vi "o3 49i Serial Data Recording & DECADEv3.2.vi"() -> ()   [LabVIEW 2014]
uses:
  <vilib>/Platform/TimedLoop/XDataNode/timing_clust.ctl
  <vilib>/Platform/TimedLoop/XDataNode/nitl_modes.ctl
  <vilib>/Platform/TimedLoop/XDataNode/wakeup.ctl
  C:/Program Files (x86)/National Instruments/LabVIEW 2014/examples/Data Communication/Network Streams/Simple Network Streams/support/Network Stream Command.ctl
  <vilib>/Utility/error.llb/whitespace.ctl
  <vilib>/Instr/_visa.llb/VISA Configure Serial Port (Instr).vi
  <vilib>/Utility/tcp.llb/UDP Multicast Write-Only Open.vi
  <vilib>/platform/TimedLoop/XDataNode/XDataNode.xnode
  <vilib>/Platform/TimedLoop/XDataNode/XDNodeRunTimeDep.lvlib
panel:
  in  "MFC_1 SLPM set value":dbl
  out "Stop File Write":bool
  out "Default file name":string
  out "error out":errorcluster
  out "V6":bool
  in  "Clear Display\nErrors":bool
  out "Data Processing":bool
  out "Serial Visa Error":errorcluster
  out "SEPTIC TCP Error Out":errorcluster
  out "TCP packet\nSend to SEPTIC":bool
  out "UDP Time Stamp Offset":i32=1
  out "Data Array":string[](array[string])
  out "UDP packet \nstatus":bool
  out "UDP_Out_Error":errorcluster
  out "FISH TCP Error Out":errorcluster
  out "TCP packet\nSend to FISH":bool
  out "TCP Binary Packet":string
  out "Scan from String Error Counter\nfrom process loop":i32
  out "Read Error Counter\nfrom process loop":i32
  in  "milliseconds to wait":u32=330
  in  "ID":string="»"
  in  "VISA resource name":refnum<visa-resource-name>="ASRL6::INSTR"
  out "Data In Array":string[](array[string])
  out "UDP_ASCII_Out":string
  out "UDP_Pack_num":u32
  out "Flight Number":string
  in  "ue9LJ temp":u16
  out "Data String":string
  out "Internal packet":string[](array[string])
  out "RAW DATA":string
  in  "stop":bool
  out "Number of Send & Read Error\nfrom Acquire Loop":i32
  out "Command In":string
  # "o3_conc"
  # "Bench_temp"
  # "pressure"
  # "cell_a_nt"
  # "cell_b_int"
  # "flow_a"
  # "flow_b"
  # "lamp_temp"
  # "flags"
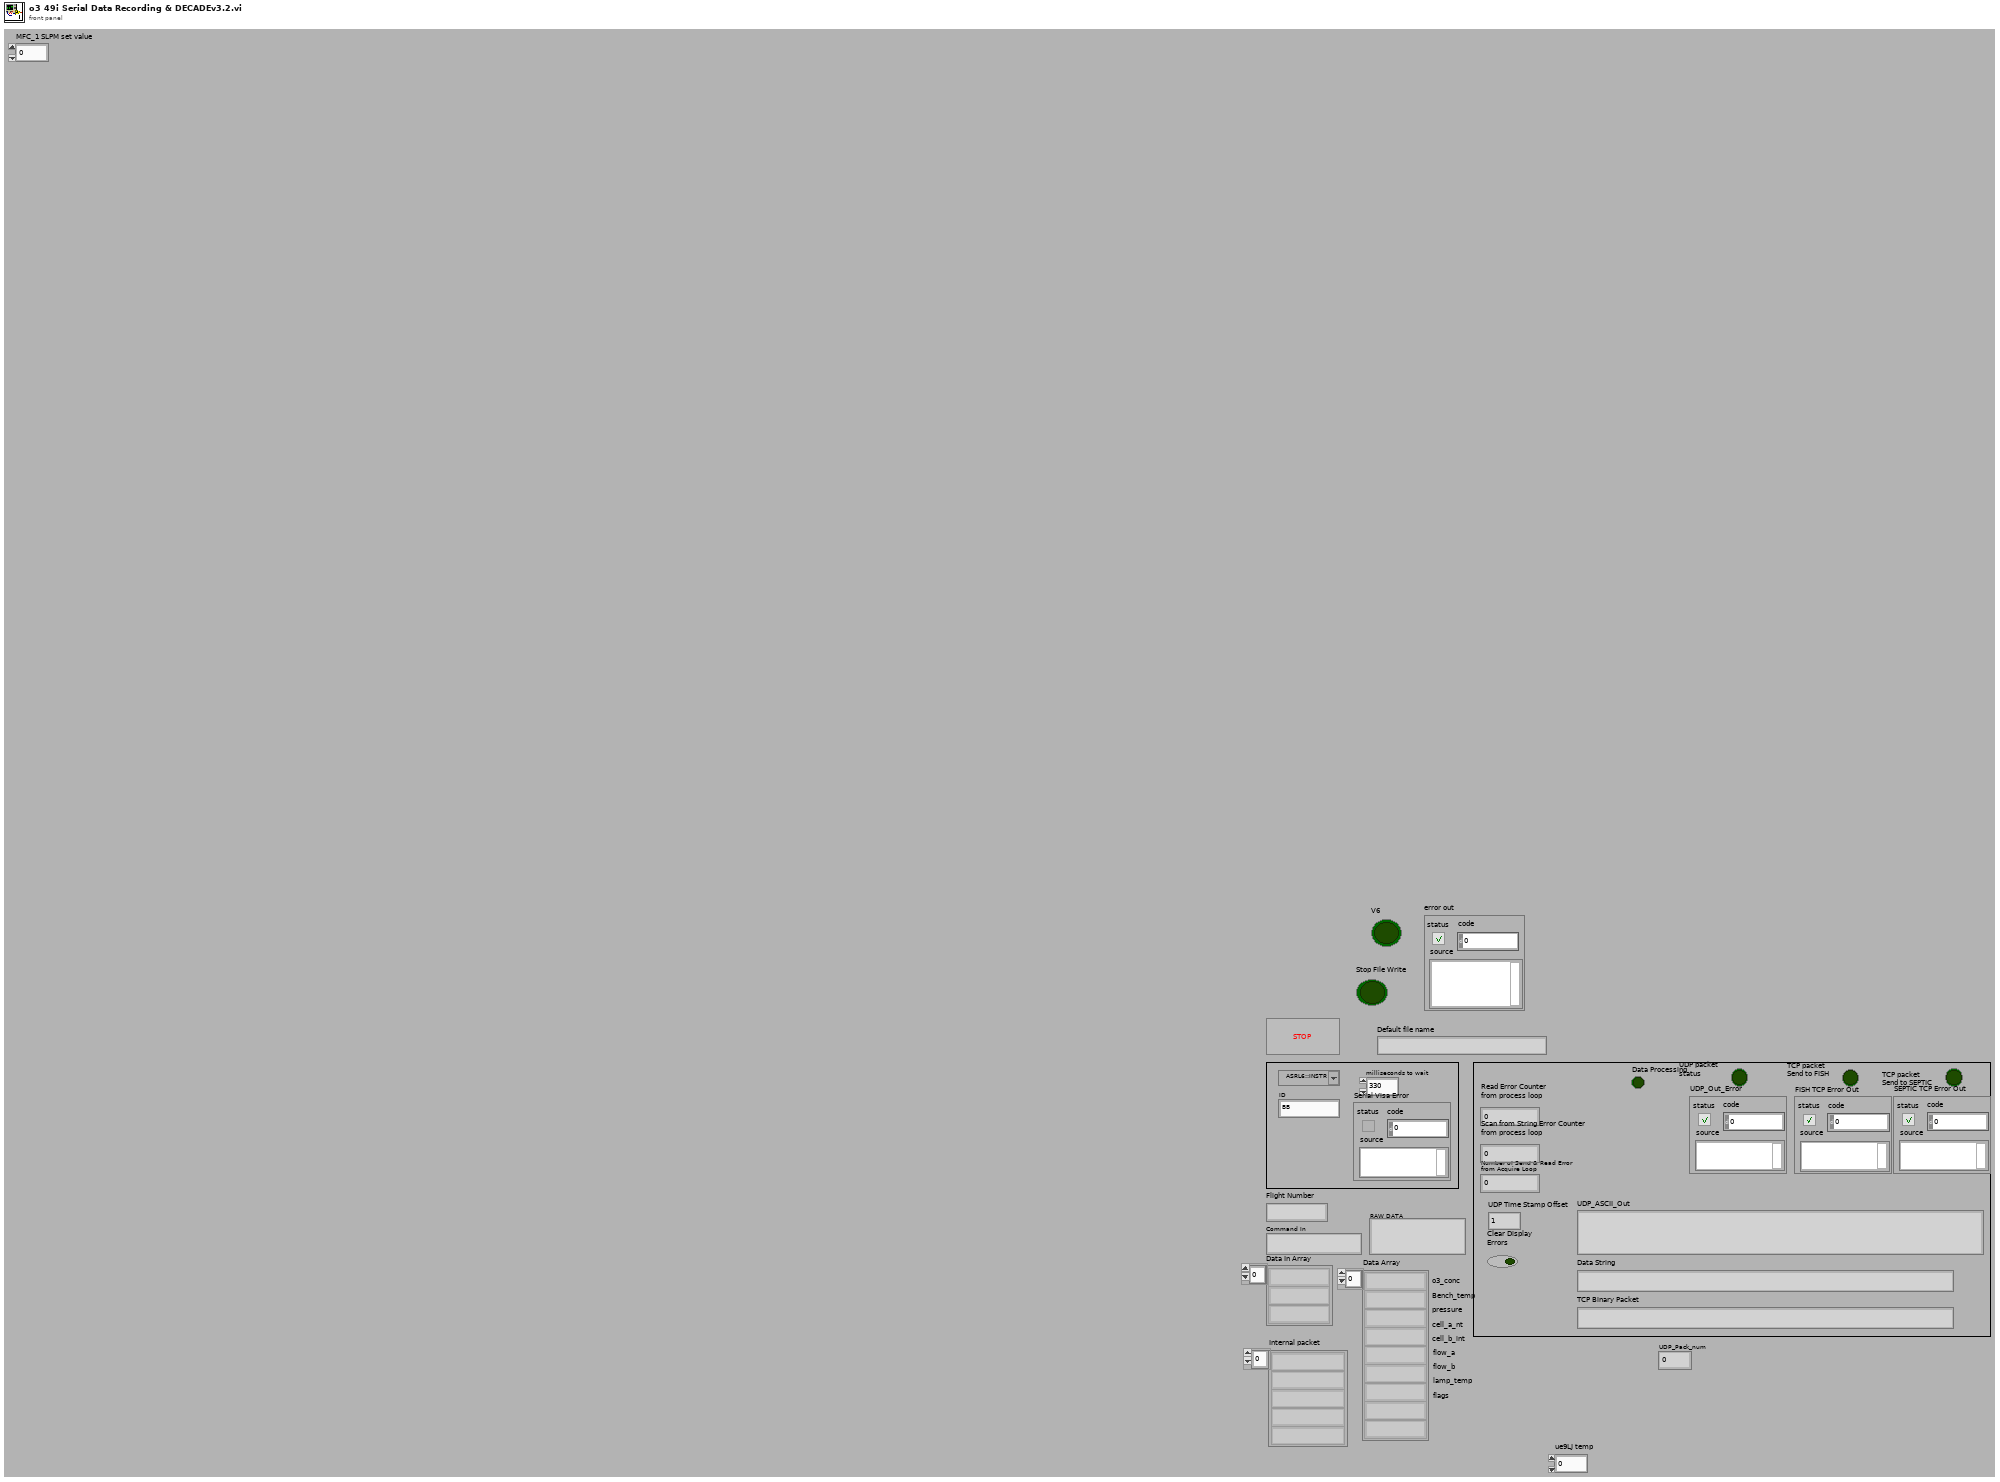
[diagram p1: front panel]
types:
  T1 = typedef "XDNodeRunTimeDep.lvlib/timing_clust.ctl" = cluster{"Expected End [f-1]":u64, "Actual End [f-1]":u64, "Finished Late? [f-1]":bool, "Expected End [i-1]":u64, "Actual End [i-1]":u64, "Finished Late? [i-1]":bool, "Expected Start [i]":u64, "Actual Start [i]":u64, "Expected Start [f]":u64, "Actual Start [f]":u64, "Source Name":string, "Structure Name":string, "Period":i64, "Deadline":i64, "Offset":i64, "Start":i64, "Priority":i32, "Timeout":i32, "Mode":T2, "Wakeup Reason":T3, "Error":errorcluster, "Source Type":string, "Secondary Source Type":string, "Global End Time":u64, "Global Start Time":u64, "Frame Duration":u64, "Iteration Duration":u64, "Assigned CPU":i32, "I/O Scan Engine Mode":u32}
  T2 = typedef "XDNodeRunTimeDep.lvlib/nitl_modes.ctl" = enum32{"No Change", "Process missed periods, maintain original phase", "Discard missed periods, maintain original phase", "Process missed periods, ignore original phase", "Discard missed periods, ignore original phase"}
  T3 = typedef "XDNodeRunTimeDep.lvlib/wakeup.ctl" = enum32{"Normal", "Aborted", "Asynchronous wakeup", "Timing source error", "Timed loop error", "Timeout"}
  T4 = typedef "Network Stream Command.ctl" = cluster{"Message":string, "Message Data":variant}
  T5 = enum16{"open", "replace", "create", "open or create", "replace or create", "replace or create with confirmation"}
  T6 = typedef "whitespace.ctl" = u16
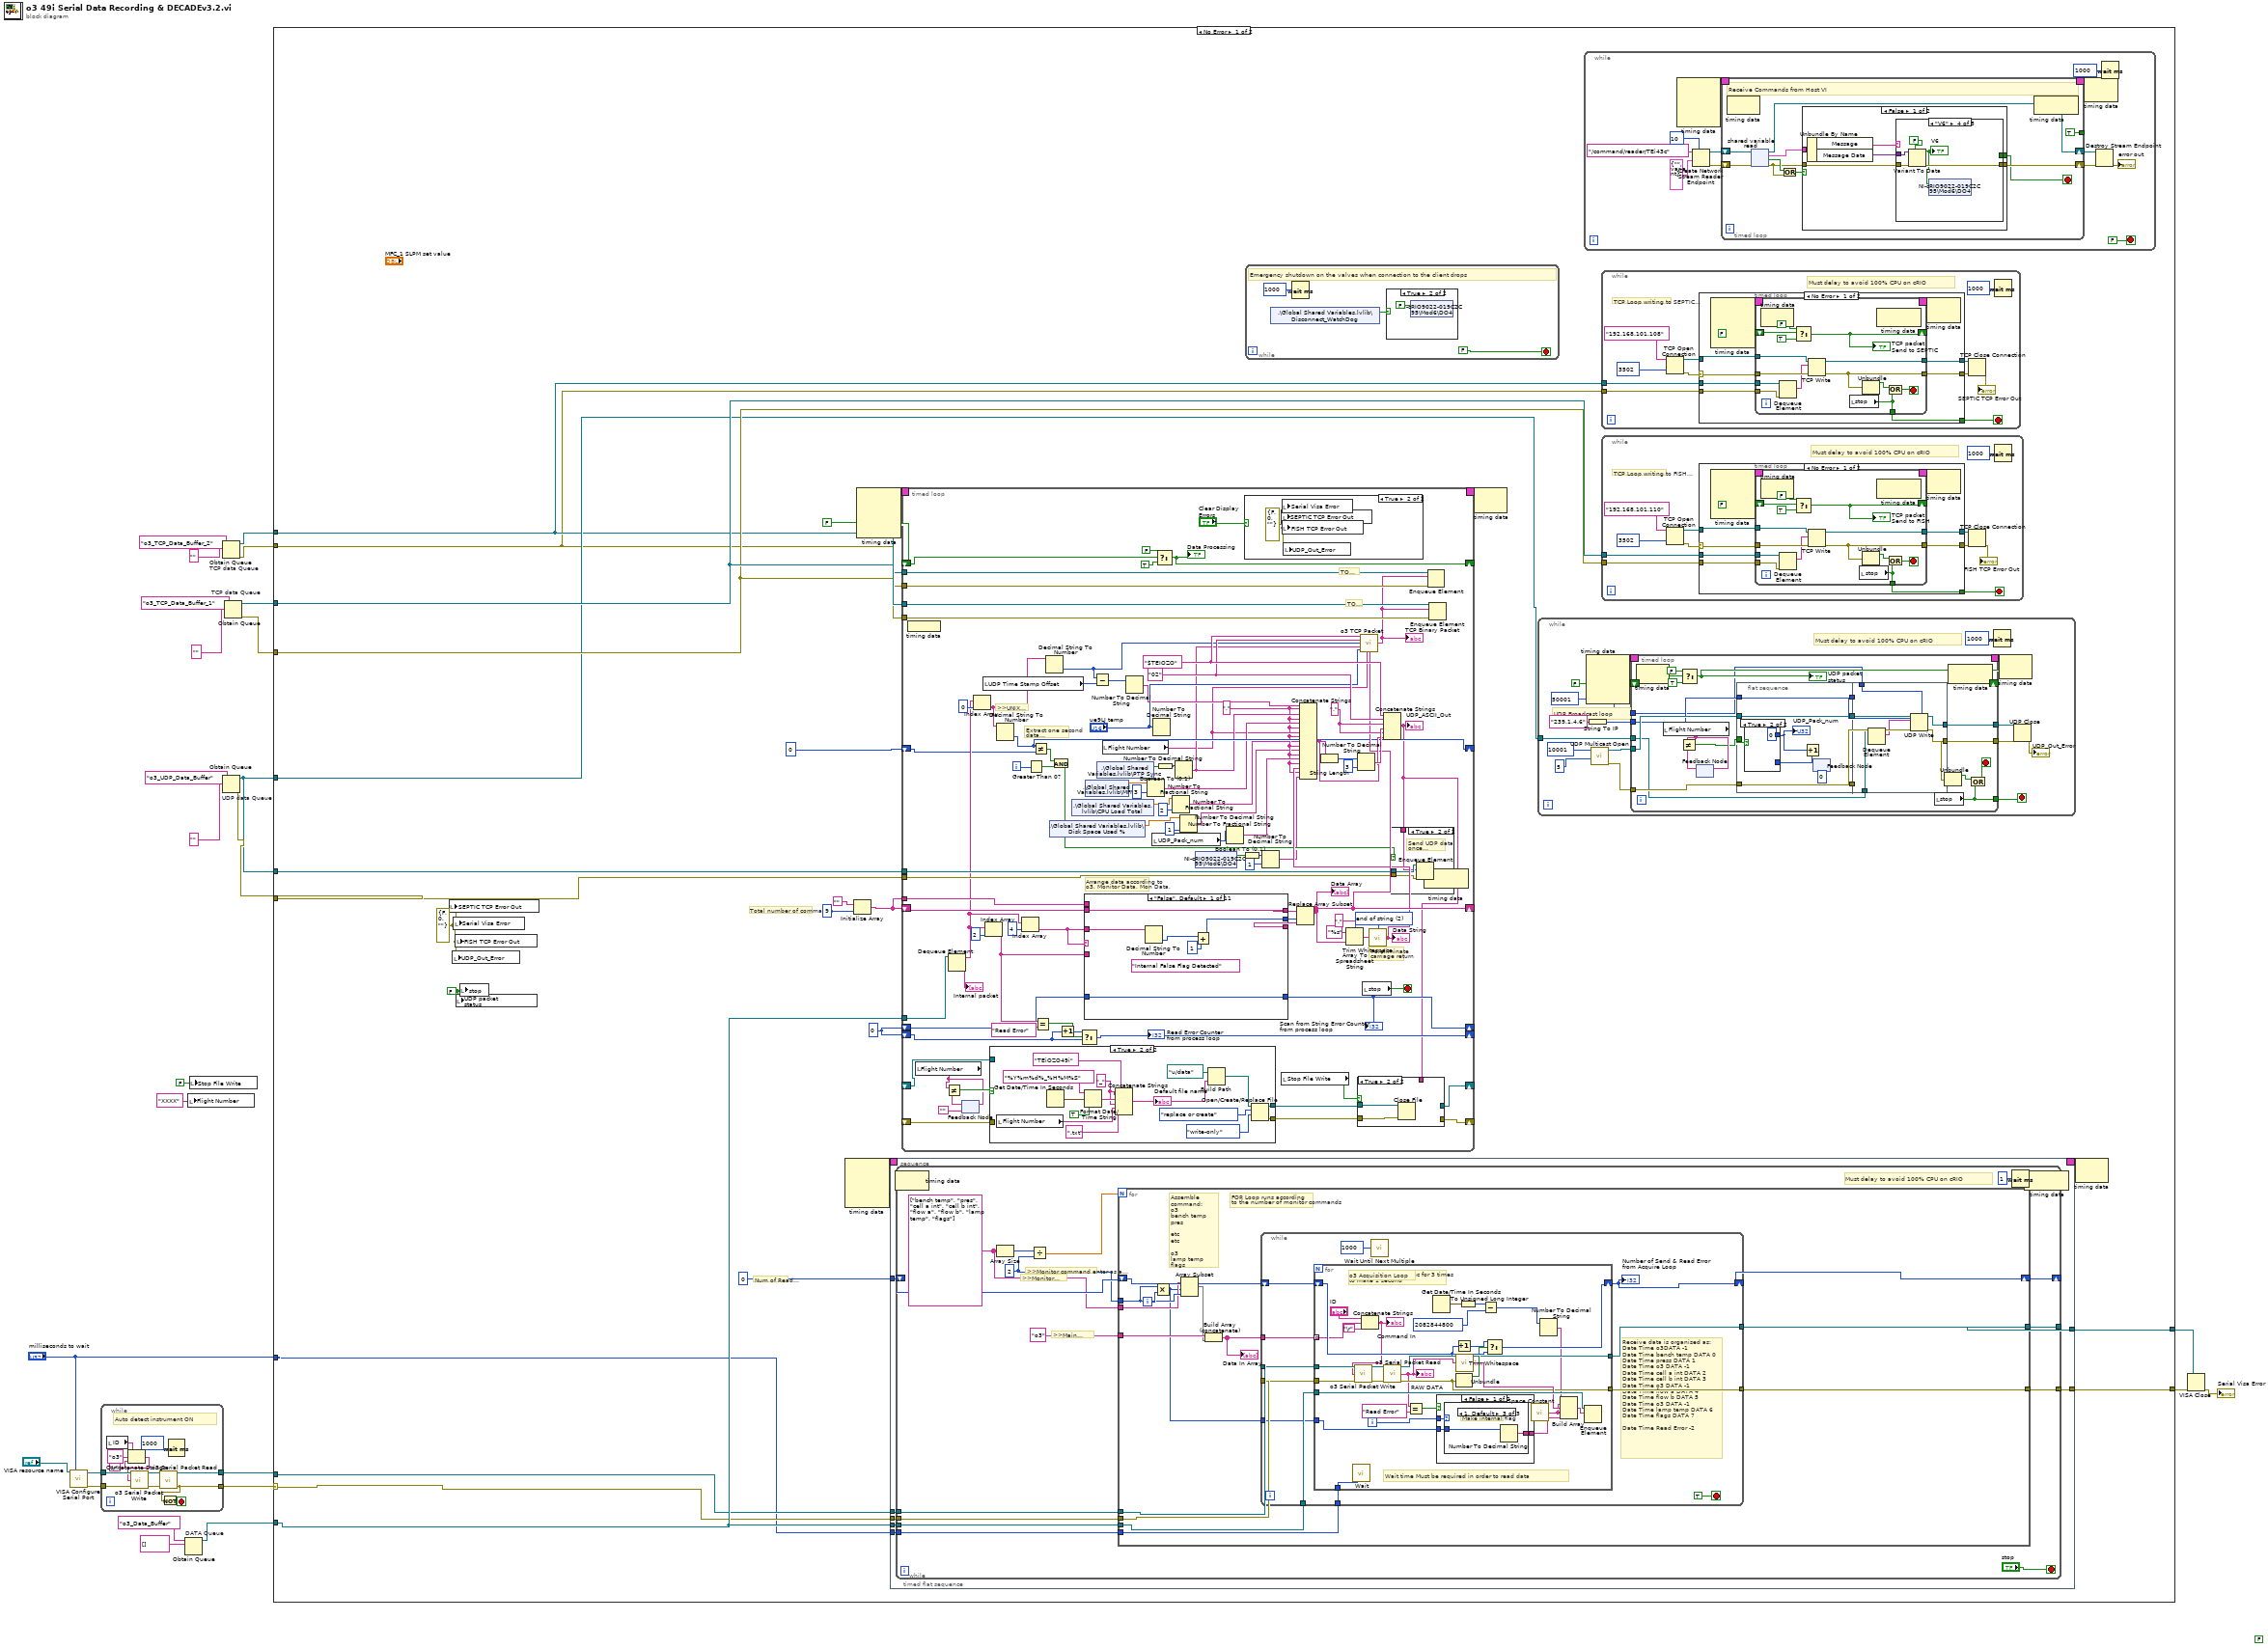
[diagram p0: block diagram]
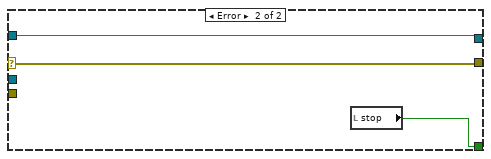
[diagram p3: hidden frame]
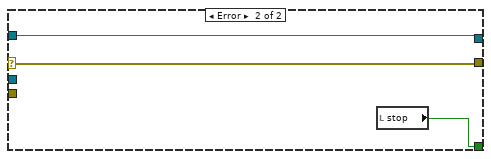
[diagram p4: hidden frame]
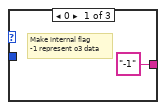
[diagram p5: hidden frame]
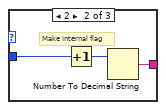
[diagram p6: hidden frame]
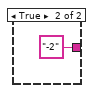
[diagram p7: hidden frame]
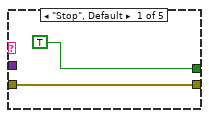
[diagram p8: hidden frame]
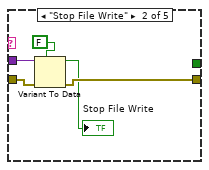
[diagram p9: hidden frame]
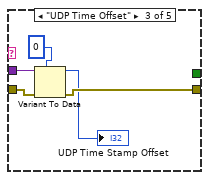
[diagram p10: hidden frame]
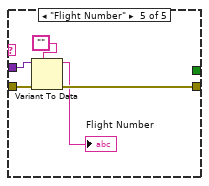
[diagram p11: hidden frame]
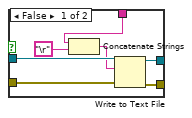
[diagram p15: hidden frame]
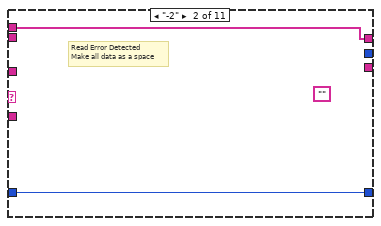
[diagram p18: hidden frame]
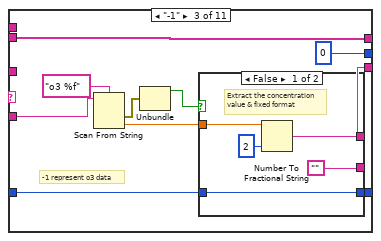
[diagram p19: hidden frame]
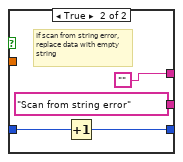
[diagram p20: hidden frame]
diagram:
  (unwired) FALSE
  n1 = call-poly "VISA Configure Serial Port"("VISA resource name"="VISA resource name", "timeout (10sec)"="milliseconds to wait") -> ("VISA resource name out"=w8:refnum<visa-resource-name>, "error out"=w7:errorcluster)  [unwired: 12 in]
  n2 = while {
    tunnel: [w36] -> w10
    tunnel: [w35] -> w9
    tunnel: w8 -> [w34]
    tunnel: w7 -> [w33]
    stop <- w37 stop-if-true
    # "Auto detect instrument ON"
    n3 = local read "ID"() -> (w31:string)
    n4 = Concatenate Strings(w31, "o3" ("string"), "\r") -> (w28:string)
    n5 = call "o3 Serial Packet Write.vi"("VISA resource name In"=w34, "Data in"=w28, "error in (no error)"=w33) -> ("VISA resource name Out"=w32:refnum<visa-resource-name>, "error out"=w38:errorcluster)  [unwired: 11 in]
    n6 = call "o3 Serial Packet Read.vi"("VISA resource In"=w32, "error in"=w38) -> ("VISA resource Out"=w35:refnum<visa-resource-name>, "error out"=w36:errorcluster)  [unwired: 11 in, 1 out]
    n7 = Not(x=w36) -> (.not. x?=w37:bool)
    n8 = Wait (ms)(milliseconds to wait=u32 1000) -> ()  [unwired: 1 out]
  }
  n9 = Obtain Queue "DATA Queue"(name (unnamed)="o3_Data_Buffer", element data type=string[] []) -> (queue out=w24:refnum<queue>)  [unwired: 3 in, 2 out]
  n10 = local write "Flight Number"("XXXX" ("Flight Number")) -> ()
  n11 = local write "Stop File Write"(FALSE ("Stop File Write")) -> ()
  n12 = Obtain Queue "TCP data Queue"(name (unnamed)="o3_TCP_Data_Buffer_2", element data type="") -> (queue out=w13:refnum<queue>, error out=w12:errorcluster)  [unwired: 3 in, 1 out]
  n13 = Obtain Queue "UDP data Queue"(name (unnamed)="o3_UDP_Data_Buffer", element data type="") -> (queue out=w14:refnum<queue>, error out=w15:errorcluster)  [unwired: 3 in, 1 out]
  n14 = Obtain Queue "TCP data Queue"(name (unnamed)="o3_TCP_Data_Buffer_1", element data type="") -> (queue out=w19:refnum<queue>, error out=w18:errorcluster)  [unwired: 3 in, 1 out]
  n15 = case shown="No Error" w10 {
    selector: w10 -> [w48 w682]
    tunnel: [w64 w682] -> w21
    tunnel: [w63 w681] -> w22
    tunnel: w24 -> [w60 _]
    tunnel: w9 -> [w47 w681]
    tunnel: w19 -> [w53 _]
    tunnel: w18 -> [w52 _]
    tunnel: w14 -> [w51 _]
    tunnel: w15 -> [w50 _]
    tunnel: w14 -> [w49 _]
    tunnel: w13 -> [w45 _]
    tunnel: w12 -> [w44 _]
    tunnel: "milliseconds to wait" -> [w43 _]
    frame No Error {
      w41 = errorcluster {"status"=FALSE, "code"=0, "source"=""} ("UDP Error Out")
      w55 = 0
      w54 = FALSE ("stop")
      # "Num of Read Error"
      # "Total number of commands"
      n16 = local write "SEPTIC TCP Error Out"(w41) -> ()
      n17 = local write "UDP_Out_Error"(w41) -> ()
      n18 = local write "Serial Visa Error"(w41) -> ()
      n19 = local write "FISH TCP Error Out"(w41) -> ()
      n20 = local write "UDP packet \nstatus"(w54) -> ()
      n21 = local write "stop"(w54) -> ()
      n22 = node-c288() -> (w40:T1)  [unwired: 4 in]
      n23 = Initialize Array("", 9) -> (w56:string[])
      n24 = node-c288() -> (w62:T1)  [unwired: 4 in]
      n25 = timed-sequence {
        timing: w40 -> [_]
        timing-out: [_] -> w39
        tunnel: [w159] -> w64
        tunnel: [w158] -> w63
        tunnel: w60 -> [w157]
        tunnel: 0 -> [w156]
        tunnel: w48 -> [w155]
        tunnel: w47 -> [w154]
        tunnel: w43 -> [w153]
        n26 = timed-flat-sequence {
          tunnel: [w166] -> w159
          tunnel: [w165] -> w158
          tunnel: w157 -> [w164]
          tunnel: w156 -> [w163]
          tunnel: w155 -> [w162]
          tunnel: w154 -> [w161]
          tunnel: w153 -> [w160]
          n27 = node-c288() -> ()  [unwired: 1 in, 1 out]
          n28 = while {
            tunnel: [w170] -> w166
            tunnel: w161 -> [w181]
            tunnel: w162 -> [w180]
            tunnel: [w179] -> w165
            tunnel: w164 -> [w178]
            shift-right: [w176] -> _
            shift-left: w163 -> [w177]
            tunnel: w160 -> [w168]
            stop <- "stop" stop-if-true
            w171 = 2
            w173 = string[] ["bench temp", "pres", "cell a int", "cell b int", "flow a", "flow b", "lamp temp", "flags"]
            # "Must delay to avoid 100% CPU on cRIO"
            # ">>Monitor command enter as a pair>>"
            # ">>Main commands>>"
            # ">>Monitor Command>>"
            n29 = Array Size(array=w173) -> (size(s)=w174:i32)
            n30 = Divide(x=w174, y=w171) -> (x/y=w172:dbl)
            n31 = for {
              N: w172 -> [_]
              tunnel: w181 -> [w189]
              tunnel: w180 -> [w188]
              tunnel: [w196] -> w170
              shift-right: [w194] -> w176
              shift-left: w177 -> [w195]
              tunnel: [w193] -> w179
              tunnel: w178 -> [w192]
              tunnel: w173 -> [w185]
              tunnel: "o3" -> [w190]
              tunnel: w171 -> [w186]
              tunnel: w168 -> [w182]
              i -> [w187]
              # "FOR Loop runs according\nto the number of monitor commands"
              # "Assemble command:\no3\nbench temp\npres\n\netc\netc\n\no3\nlamp temp\nflags"
              n32 = Multiply(x=w186, y=w187) -> (x*y=w183:i32)
              n33 = Array Subset(array=w185, index=w183, length=w186) -> (w184:string[])
              n34 = Build Array (concatenate)(w190, w184) -> (w191:string[])
              "Data In Array" <- w191
              n35 = while {
                tunnel: [w208] -> w196
                tunnel: w191 -> [w206]
                tunnel: [w204] -> w193
                tunnel: w192 -> [w203]
                tunnel: w188 -> [w202]
                tunnel: w189 -> [w201]
                tunnel: w183 -> [w200]
                shift-right: [w205] -> w194
                shift-left: w195 -> [w207]
                tunnel: w182 -> [w197]
                stop <- TRUE stop-if-true
                # "Receive data is organised as:\nDate Time o3DATA -1\nDate Time bench temp DATA 0\nDate Time press DATA 1\nDate Time o3 DATA -1\nDate Time cell a int DATA 2\nDate Time cell b int DATA 3\nDate Time o3 DATA -1\nDate Time flow a DATA 4\nDate Time flow b DATA 5\nDate Time o3 DATA -1\nDate Time lamp temp DATA 6\nDate Time flags DATA 7\n\nDate Time Read Error -2"
                n36 = for {
                  tunnel: w202 -> [w225]
                  tunnel: [w226] -> w208
                  tunnel: w206 -> [w223] mode=indexing
                  tunnel: [w227] -> w204
                  tunnel: w203 -> [w233]
                  tunnel: w201 -> [w228]
                  tunnel: w200 -> [w222]
                  shift-right: [w237] -> w205
                  shift-left: w207 -> [w238]
                  tunnel: w197 -> [w211]
                  i -> [w215]
                  # "Wait time Must be required in order to read data"
                  # "Acquire every 330msec for 3 times\nto make 1 second"
                  # "o3 Acquisition Loop"
                  n37 = call "Wait"("Count(mSec)"=w211) -> ()  [unwired: 1 out]
                  n38 = Concatenate Strings("ID", w223, "\r") -> (w221:string)
                  "Command In" <- w221
                  n39 = call "o3 Serial Packet Write.vi"("VISA resource name In"=w228, "Data in"=w221, "error in (no error)"=w225) -> ("VISA resource name Out"=w230:refnum<visa-resource-name>, "error out"=w229:errorcluster)  [unwired: 11 in]
                  n40 = call "o3 Serial Packet Read.vi"("VISA resource In"=w230, "error in"=w229) -> ("VISA resource Out"=w227:refnum<visa-resource-name>, "Data Out"=w218:string, "error out"=w226:errorcluster)  [unwired: 11 in]
                  "RAW DATA" <- w218
                  n41 = Equal?(x=w218, y="Read Error") -> (x = y?=w216:bool)
                  n42 = Get Date/Time In Seconds() -> (seconds since 1Jan1904=w210:timestamp)
                  n43 = case shown="False" w216 {
                    tunnel: [w241 "-2"] -> w231
                    tunnel: w215 -> [w240 _]
                    tunnel: w222 -> [w239 _]
                    frame False {
                      n44 = case shown="1, Default" w240 {
                        tunnel: ["-1" w245 w247] -> w241
                        tunnel: w239 -> [_ w243 w246]
                        frame 0 {
                          # "Make internal flag\n-1 represent o3 data"
                        }
                        frame 2 {
                          # "Make internal flag"
                          n45 = Increment(x=w243) -> (x+1=w244:i32)
                          n46 = Number To Decimal String(number=w244) -> (decimal integer string=w245:string)  [unwired: 1 in]
                        }
                        frame 1, Default {
                          # "Make internal flag"
                          n47 = Number To Decimal String(number=w246) -> (decimal integer string=w247:string)  [unwired: 1 in]
                        }
                      }
                    }
                    frame True {
                    }
                  }
                  n48 = Increment(x=w238) -> (x+1=w234:i32)
                  n49 = Unbundle(w226) -> ("status"=w235:bool)  [unwired: 2 out]
                  n50 = call <vilib>:"Trim Whitespace.vi"("string"=w218) -> ("trimmed string"=w232:string)  [unwired: 1 in]
                  n51 = To Unsigned Long Integer(number=w210) -> (unsigned 32bit integer=w214:u32)
                  n52 = Subtract(x=w214, y=u32 2082844800) -> (x-y=w209:u32)
                  n53 = Select(t=w234, s=w235, f=w238) -> (s? t:f=w237:i32)
                  n54 = call <vilib>:"Space Constant.vi"() -> ("String"=w219:string)
                  n55 = Number To Decimal String(number=w209) -> (decimal integer string=w212:string)  [unwired: 1 in]
                  n56 = Build Array(w212, w219, w232, w219, w231) -> (w220:string[])
                  n57 = Enqueue Element(queue=w233, element=w220) -> ()  [unwired: 2 in, 3 out]
                }
                "Number of Send & Read Error\nfrom Acquire Loop" <- w205
                n58 = call "Wait Until Next Multiple"("Count(mSec)"=u32 1000) -> ()  [unwired: 1 out]
              }
            }
            n59 = Wait (ms)(milliseconds to wait=u32 1) -> ()  [unwired: 1 out]
          }
          n60 = node-c288() -> ()  [unwired: 1 in, 1 out]
        }
      }
      n61 = timed-loop {
        timing: w62 -> [_]
        timing-out: [_] -> w61
        tunnel: w60 -> [w455]
        shift-right: [w423] -> _
        shift-left: w56 -> [w444]
        shift-right: [w432] -> _
        shift-left: w55 -> [w429]
        tunnel: w56 -> [w431]
        shift-right: [w427] -> _
        shift-left: w55 -> [w428]
        tunnel: w53 -> [w422]
        tunnel: w52 -> [w421]
        tunnel: w51 -> [w419]
        tunnel: w50 -> [w418]
        shift-right: [w410] -> _
        shift-left: 0 -> [w413]
        tunnel: w45 -> [w408]
        tunnel: w44 -> [w407]
        shift-right: [w399] -> _
        shift-left: FALSE -> [w402]
        shift-right: [w396] -> _
        shift-left: _ -> [w388]
        shift-right: [w386] -> _
        shift-left: _ -> [w387]
        i -> [w411]
        stop <- w453 stop-if-true
        w437 = T6 2 items=["both", "start of string", "end of string"] ("location (both)")
        w373 = ","
        w425 = "02"
        w446 = ","
        w426 = "$TEIOZO"
        # "TO SEPTIC"
        # "TO FISH"
        # "Extract one second data\nfor UDP sending"
        # "Arrange data according to\no3, Monitor Data, Mon Data,"
        # "To eliminate\ncarriage return"
        # ">>UNIX TIME>>"
        n62 = node-c288() -> ()  [unwired: 1 in]
        n63 = local read "Flight Number"() -> (w391:string)
        n64 = Dequeue Element(queue=w455) -> (element=w416:string[])  [unwired: 2 in, 3 out]
        "Internal packet" <- w416
        n65 = feedback #1("" ("Flight Number")) -> (w393:string)
        n66 = Not Equal?(x=w391, y=w393) -> (x != y?=w392:bool)
        n67 = feedback-in #1(w391) -> ()
        n68 = Index Array(array=w416, index=0) -> (element=w415:string)
        n69 = local read "UDP Time Stamp Offset"() -> (w368:i32)
        n70 = Index Array(array=w416, index=2) -> (element=w435:string)
        n71 = case shown="True" w392 {
          tunnel: [w457 w459] -> w390
          tunnel: [w456 w458] -> w389
          tunnel: w388 -> [w457 _]
          tunnel: w387 -> [w456 _]
          frame False {
          }
          frame True {
            w466 = "_" ("string")
            n72 = local read "Flight Number"() -> (w472:string)
            n73 = Get Date/Time In Seconds() -> (seconds since 1Jan1904=w467:timestamp)
            n74 = Format Date/Time String(time format string (%c)="%Y%m%d%_%H%M%S", seconds (now)=w467, UTC format=TRUE) -> (date/time string=w470:string)
            n75 = Concatenate Strings("TEiOZO49i" ("string"), w466, w470, w466, w472, ".txt" ("string")) -> (w464:string)
            "Default file name" <- w464
            n76 = Build Path(base path=path "u:/data", name or relative path=w464) -> (appended path=w460:path)
            n77 = Open/Create/Replace File(file path (use dialog)=w460, operation (0:open)=T5."replace or create", access (0:read/write)=enum16{"read/write", "read-only", "write-only"}."write-only") -> (refnum out=w459:refnum<file>, error out=w458:errorcluster)  [unwired: 3 in, 1 out]
          }
        }
        n78 = Decimal String To Number(string=w415) -> (number=w410:i32)  [unwired: 2 in, 1 out]
        n79 = Index Array(array=w416, index=4) -> (element=w443:string)
        n80 = Greater Than 0?(x=w411) -> (x > 0?=w414:bool)
        n81 = Not Equal?(x=w410, y=w413) -> (x != y?=w412:bool)
        n82 = Equal?(x=w435, y="Read Error") -> (x = y?=w433:bool)
        n83 = Decimal String To Number(string=w415) -> (number=w404:i32)  [unwired: 2 in, 1 out]
        n84 = shared-variable ".\\Global Shared Variables.lvlib\\Disk Space Used %"() -> (w370:dbl)  [unwired: 1 in, 1 out]
        n85 = Compound Arithmetic op=AND(w412, w414) -> (w409:bool)
        n86 = Increment(x=w429) -> (x+1=w430:i32)
        n87 = shared-variable ".\\Global Shared Variables.lvlib\\CPU Load Total"() -> (w385:dbl)  [unwired: 1 in, 1 out]
        n88 = Select(t=w430, s=w433, f=w429) -> (s? t:f=w432:i32)
        "Read Error Counter\nfrom process loop" <- w432
        n89 = case shown="\"False\", Default" w443 {
          tunnel: w443 -> [w490 _ _ w523 w542 w563 w584 w605 w626 w647 w668]
          tunnel: w444 -> [w491 _ w503 w524 w543 w564 w585 w606 w627 w648 w669]
          tunnel: w435 -> [_ _ w500 w519 w538 w560 w581 w602 w623 w644 w665]
          tunnel: [w491 w493 w503 w524 w543 w564 w585 w606 w627 w648 w669] -> w442
          tunnel: [w488 _ 0 ("index") w521 w540 w561 w582 w603 w624 w645 w666] -> w441
          tunnel: [_ _ w498 w517 w536 w559 w580 w601 w622 w643 w660] -> w440
          tunnel: w431 -> [_ w493 _ _ _ _ _ _ _ _ _]
          tunnel: w428 -> [w486 w492 w495 w514 w533 w554 w575 w596 w617 w638 w659]
          tunnel: [w486 w492 w494 w513 w532 w553 w574 w595 w616 w637 w658] -> w427
          frame "False", Default {
            (unwired) "Internal False Flag Detected"
            n90 = Decimal String To Number(string=w490) -> (number=w487:i32)  [unwired: 2 in, 1 out]
            n91 = Add(x=w487, y=1) -> (x+y=w488:i32)
          }
          frame "-2" {
            (unwired) ""
            # "Read Error Detected\nMake all data as a space"
          }
          frame "-1" {
            # "-1 represent o3 data"
            n92 = Scan From String(format string="o3 %f", input string=w500) -> (error out=w497:errorcluster, output 1=w499:dbl)  [unwired: 3 in, 2 out]
            n93 = Unbundle(w497) -> ("status"=w496:bool)  [unwired: 2 out]
            n94 = case shown="False" w496 {
              tunnel: w499 -> [w508 _]
              tunnel: [w507 ""] -> w498
              tunnel: w495 -> [w506 w511]
              tunnel: [w506 w510] -> w494
              tunnel: ["" "Scan from string error"] -> _
              frame False {
                # "Extract the concentration\nvalue & fixed format"
                n95 = Number To Fractional String(number=w508, precision (6)=i16 2) -> (F-format string=w507:string)  [unwired: 2 in]
              }
              frame True {
                # "If scan from string error,\nreplace data with empty\nstring"
                n96 = Increment(x=w511) -> (x+1=w510:i32)
              }
            }
          }
          frame "0" {
            # "0 represents bench temp data; bench temp 022.6 deg C, actual 022.7"
            n97 = Scan From String(format string="%[^,], %s %f ", input string=w519) -> (error out=w516:errorcluster, output 3=w518:dbl)  [unwired: 7 in, 2 out]
            n98 = Decimal String To Number(string=w523) -> (number=w522:i32)  [unwired: 2 in, 1 out]
            n99 = Unbundle(w516) -> ("status"=w515:bool)  [unwired: 2 out]
            n100 = case shown="False" w515 {
              tunnel: w518 -> [w528 _]
              tunnel: [w527 ""] -> w517
              tunnel: w514 -> [w526 w530]
              tunnel: [w526 w529] -> w513
              frame False {
                # "Extract the actual value\n& fixed format"
                n101 = Number To Fractional String(number=w528, precision (6)=i16 1) -> (F-format string=w527:string)  [unwired: 2 in]
              }
              frame True {
                (unwired) "Scan from string error"
                # "If scan from string error,\nreplace data with empty\nstring"
                n102 = Increment(x=w530) -> (x+1=w529:i32)
              }
            }
            n103 = Increment(x=w522) -> (x+1=w521:i32)
          }
          frame "1" {
            # "1 represents pres data; pres 725.3 mmHg, actual 725.4"
            n104 = Scan From String(format string="%[^,], %s %f ", input string=w538) -> (error out=w535:errorcluster, output 3=w537:dbl)  [unwired: 7 in, 2 out]
            n105 = Decimal String To Number(string=w542) -> (number=w541:i32)  [unwired: 2 in, 1 out]
            n106 = Unbundle(w535) -> ("status"=w534:bool)  [unwired: 2 out]
            n107 = case shown="False" w534 {
              tunnel: w537 -> [w548 _]
              tunnel: [w547 ""] -> w536
              tunnel: w533 -> [w546 w551]
              tunnel: [w546 w550] -> w532
              tunnel: ["" "Scan from string error"] -> _
              frame False {
                # "Extract the actual value\n& fixed format"
                n108 = Number To Fractional String(number=w548, precision (6)=i16 1) -> (F-format string=w547:string)  [unwired: 2 in]
              }
              frame True {
                # "If scan from string error,\nreplace data with empty\nstring"
                n109 = Increment(x=w551) -> (x+1=w550:i32)
              }
            }
            n110 = Increment(x=w541) -> (x+1=w540:i32)
          }
          frame "2" {
            # "2 represents cell a int data; cell a int 63246 Hz"
            n111 = Scan From String(format string="cell a int %d", input string=w560) -> (error out=w556:errorcluster, output 1=w557:i32)  [unwired: 3 in, 2 out]
            n112 = Decimal String To Number(string=w563) -> (number=w562:i32)  [unwired: 2 in, 1 out]
            n113 = Unbundle(w556) -> ("status"=w555:bool)  [unwired: 2 out]
            n114 = case shown="False" w555 {
              tunnel: [w569 ""] -> w559
              tunnel: w557 -> [w568 _]
              tunnel: w554 -> [w567 w572]
              tunnel: [w567 w571] -> w553
              tunnel: ["" "Scan from string error"] -> _
              frame False {
                # "Extract the actual value\n& fixed format"
                n115 = Number To Fractional String(number=w568, precision (6)=i16 0) -> (F-format string=w569:string)  [unwired: 2 in]
              }
              frame True {
                # "If scan from string error,\nreplace data with empty\nstring"
                n116 = Increment(x=w572) -> (x+1=w571:i32)
              }
            }
            n117 = Increment(x=w562) -> (x+1=w561:i32)
          }
          frame "3" {
            # "3 represents cell b int data; cell b int 63246 Hz"
            n118 = Scan From String(format string="cell b int %d", input string=w581) -> (error out=w577:errorcluster, output 1=w578:i32)  [unwired: 3 in, 2 out]
            n119 = Decimal String To Number(string=w584) -> (number=w583:i32)  [unwired: 2 in, 1 out]
            n120 = Unbundle(w577) -> ("status"=w576:bool)  [unwired: 2 out]
            n121 = case shown="False" w576 {
              tunnel: [w590 ""] -> w580
              tunnel: w578 -> [w589 _]
              tunnel: w575 -> [w588 w593]
              tunnel: [w588 w592] -> w574
              tunnel: ["" "Scan from string error"] -> _
              frame False {
                # "Extract the actual value\n& fixed format"
                n122 = Number To Fractional String(number=w589, precision (6)=i16 0) -> (F-format string=w590:string)  [unwired: 2 in]
              }
              frame True {
                # "If scan from string error,\nreplace data with empty\nstring"
                n123 = Increment(x=w593) -> (x+1=w592:i32)
              }
            }
            n124 = Increment(x=w583) -> (x+1=w582:i32)
          }
          frame "4" {
            # "4 represents flow a data; flow a 0.696 l/m"
            n125 = Scan From String(format string="flow a %f", input string=w602) -> (error out=w598:errorcluster, output 1=w599:dbl)  [unwired: 3 in, 2 out]
            n126 = Decimal String To Number(string=w605) -> (number=w604:i32)  [unwired: 2 in, 1 out]
            n127 = Unbundle(w598) -> ("status"=w597:bool)  [unwired: 2 out]
            n128 = case shown="False" w597 {
              tunnel: [w611 ""] -> w601
              tunnel: w599 -> [w610 _]
              tunnel: w596 -> [w609 w614]
              tunnel: [w609 w613] -> w595
              tunnel: ["" "Scan from string error"] -> _
              frame False {
                # "Extract the actual value\n& fixed format"
                n129 = Number To Fractional String(number=w610, precision (6)=i16 3) -> (F-format string=w611:string)  [unwired: 2 in]
              }
              frame True {
                # "If scan from string error,\nreplace data with empty\nstring"
                n130 = Increment(x=w614) -> (x+1=w613:i32)
              }
            }
            n131 = Increment(x=w604) -> (x+1=w603:i32)
          }
          frame "5" {
            # "5 represents flow b data; flow b 0.696 l/m"
            n132 = Scan From String(format string="flow b %f", input string=w623) -> (error out=w619:errorcluster, output 1=w620:dbl)  [unwired: 3 in, 2 out]
            n133 = Decimal String To Number(string=w626) -> (number=w625:i32)  [unwired: 2 in, 1 out]
            n134 = Unbundle(w619) -> ("status"=w618:bool)  [unwired: 2 out]
            n135 = case shown="False" w618 {
              tunnel: [w632 ""] -> w622
              tunnel: w620 -> [w631 _]
              tunnel: w617 -> [w630 w635]
              tunnel: [w630 w634] -> w616
              tunnel: ["" "Scan from string error"] -> _
              frame False {
                # "Extract the actual value\n& fixed format"
                n136 = Number To Fractional String(number=w631, precision (6)=i16 3) -> (F-format string=w632:string)  [unwired: 2 in]
              }
              frame True {
                # "If scan from string error,\nreplace data with empty\nstring"
                n137 = Increment(x=w635) -> (x+1=w634:i32)
              }
            }
            n138 = Increment(x=w625) -> (x+1=w624:i32)
          }
          frame "6" {
            # "6 represents lamp temp data; lamp temp 056.1 deg C"
            n139 = Scan From String(format string="lamp temp %f", input string=w644) -> (error out=w640:errorcluster, output 1=w641:dbl)  [unwired: 3 in, 2 out]
            n140 = Decimal String To Number(string=w647) -> (number=w646:i32)  [unwired: 2 in, 1 out]
            n141 = Unbundle(w640) -> ("status"=w639:bool)  [unwired: 2 out]
            n142 = case shown="False" w639 {
              tunnel: [w653 ""] -> w643
              tunnel: w641 -> [w652 _]
              tunnel: w638 -> [w651 w656]
              tunnel: [w651 w655] -> w637
              tunnel: ["" "Scan from string error"] -> _
              frame False {
                # "Extract the actual value\n& fixed format"
                n143 = Number To Fractional String(number=w652, precision (6)=i16 1) -> (F-format string=w653:string)  [unwired: 2 in]
              }
              frame True {
                # "If scan from string error,\nreplace data with empty\nstring"
                n144 = Increment(x=w656) -> (x+1=w655:i32)
              }
            }
            n145 = Increment(x=w646) -> (x+1=w645:i32)
          }
          frame "7" {
            # "7 represents flags data; flags 1c100000"
            n146 = Scan From String(format string="flags %s", input string=w665) -> (error out=w663:errorcluster, output 1=w661:string)  [unwired: 3 in, 2 out]
            n147 = Decimal String To Number(string=w668) -> (number=w667:i32)  [unwired: 2 in, 1 out]
            n148 = Unbundle(w663) -> ("status"=w662:bool)  [unwired: 2 out]
            n149 = case shown="False" w662 {
              tunnel: w661 -> [w672 _]
              tunnel: [w672 ""] -> w660
              tunnel: w659 -> [w671 w675]
              tunnel: [w671 w674] -> w658
              tunnel: ["" "Scan from string error"] -> _
              frame False {
                # "Extract the actual value\n& fixed format"
              }
              frame True {
                # "If scan from string error,\nreplace data with empty\nstring"
                n150 = Increment(x=w675) -> (x+1=w674:i32)
              }
            }
            n151 = Increment(x=w667) -> (x+1=w666:i32)
          }
        }
        "Scan from String Error Counter\nfrom process loop" <- w427
        n152 = shared-variable ".\\Global Shared Variables.lvlib\\MFM"() -> (w384:dbl)  [unwired: 1 in, 1 out]
        n153 = Subtract(x=w404, y=w368) -> (x-y=w405:i32)
        n154 = shared-variable ".\\Global Shared Variables.lvlib\\PTP Sync"() -> (w380:bool)  [unwired: 1 in, 1 out]
        n155 = local read "Flight Number"() -> (w374:string)
        n156 = Number To Decimal String(number=w405) -> (decimal integer string=w403:string)  [unwired: 1 in]
        n157 = Number To Fractional String(number=w384, precision (6)=i16 3) -> (F-format string=w379:string)  [unwired: 2 in]
        n158 = local read "UDP_Pack_num"() -> (w451:u32)
        n159 = Number To Decimal String(number="ue9LJ temp") -> ()  [unwired: 1 in, 1 out]
        n160 = Select(t=FALSE, s=w402, f=TRUE) -> (s? t:f=w399:bool)
        "Data Processing" <- w399
        n161 = Boolean To (0,1)(Boolean=w380) -> (0, 1=w381:i16)
        n162 = Number To Fractional String(number=w385, precision (6)=i16 2) -> (F-format string=w372:string)  [unwired: 2 in]
        n163 = Number To Decimal String(number=w381) -> (decimal integer string=w375:string)  [unwired: 1 in]
        n164 = Number To Fractional String(number=w370, precision (6)=i16 1) -> (F-format string=w369:string)  [unwired: 2 in]
        n165 = shared-variable "NI-cRIO9022-019C2C95\\Mod6\\DO4"() -> (w376:bool)  [unwired: 1 in, 1 out]
        n166 = Number To Decimal String(number=w451) -> (decimal integer string=w450:string)  [unwired: 1 in]
        n167 = Boolean To (0,1)(Boolean=w376) -> (0, 1=w378:i16)
        n168 = case shown="True" "Clear Display\nErrors" {
          frame False {
          }
          frame True {
            w482 = errorcluster {"status"=FALSE, "code"=0, "source"=""} ("UDP Error Out")
            n169 = local write "SEPTIC TCP Error Out"(w482) -> ()
            n170 = local write "Serial Visa Error"(w482) -> ()
            n171 = local write "FISH TCP Error Out"(w482) -> ()
            n172 = local write "UDP_Out_Error"(w482) -> ()
          }
        }
        n173 = Number To Decimal String(number=w378, width (-)=i16 1) -> (decimal integer string=w377:string)
        n174 = local read "Stop File Write"() -> (w395:bool)
        n175 = Replace Array Subset(array=w442, new element=w440, index=w441) -> (w423:string[])
        "Data Array" <- w423
        n176 = Array To Spreadsheet String(delimiter (Tab)=",", array=w423, 3:"%s" ("format string")) -> (spreadsheet string=w436:string)
        n177 = call "o3 TCP Packet.vi"("ID"=w426, "Version"=w425, "utc_time"=w404, "PTP Sync"=w375, "ue9LJ temp"="ue9LJ temp", "Flight Number"=w374, "Data Array"=w423) -> ("TCP Binary Packet"=w406:string)  [unwired: 8 in]
        "TCP Binary Packet" <- w406
        n178 = local read "stop"() -> (w453:bool)
        n179 = call <vilib>:"Trim Whitespace.vi"("string"=w436, "location (both)"=w437) -> ("trimmed string"=w420:string)
        "Data String" <- w420
        n180 = Concatenate Strings(w403, w373, w375, w373, w379, w373, w374, w373, w372, w373, w369, w373, w450, w373, w420, w373, w377) -> (w445:string)
        n181 = String Length(string=w445) -> (length=w449:i32)
        n182 = Number To Decimal String(number=w449, width (-)=i16 3) -> (decimal integer string=w447:string)
        n183 = Concatenate Strings(w426, w425, w446, w447, w446, w445) -> (w397:string)
        "UDP_ASCII_Out" <- w397
        n184 = case shown="True" w395 {
          tunnel: w390 -> [w479 w481]
          tunnel: w389 -> [w478 w480]
          tunnel: [w475 _] -> w396
          tunnel: w397 -> [w474 _]
          tunnel: [w473 _] -> w386
          frame False {
            n185 = Concatenate Strings(w474, "\r") -> (w476:string)
            n186 = Write to Text File(file (use dialog)=w479, text=w476, error in=w478) -> (refnum out=w475:refnum<file>, error out=w473:errorcluster)  [unwired: 2 out]
          }
          frame True {
            n187 = Close File(refnum=w481, error in=w480) -> ()  [unwired: 2 out]
          }
        }
        n188 = case shown="True" w409 {
          tunnel: w419 -> [_ w485]
          tunnel: w418 -> [_ w484]
          tunnel: w397 -> [_ w483]
          frame False {
          }
          frame True {
            # "Send UDP data once\na second"
            n189 = Enqueue Element(queue=w485, element=w483, error in (no error)=w484) -> ()  [unwired: 1 in, 3 out]
          }
        }
        n190 = node-c288() -> ()  [unwired: 1 in, 1 out]
        n191 = Enqueue Element(queue=w408, element=w406, error in (no error)=w407) -> ()  [unwired: 1 in, 3 out]
        n192 = Enqueue Element(queue=w422, element=w406, error in (no error)=w421) -> ()  [unwired: 1 in, 3 out]
      }
      n193 = while {
        stop <- FALSE stop-if-true
        # "Emergency shutdown on the valves when connection to the client drops"
        n194 = shared-variable ".\\Global Shared Variables.lvlib\\Disconnect_WatchDog"() -> (w65:bool)  [unwired: 1 in, 1 out]
        n195 = Wait (ms)(milliseconds to wait=u32 1000) -> ()  [unwired: 1 out]
        n196 = case shown="True" w65 {
          frame False {
          }
          frame True {
            n197 = shared-variable "NI-cRIO9022-019C2C95\\Mod6\\DO4"(FALSE) -> ()  [unwired: 1 in, 1 out]
          }
        }
      }
      n198 = node-c288(w61) -> ()  [unwired: 1 out]
      n199 = while {
        tunnel: w49 -> [w310]
        stop <- w311 stop-if-true
        # "Must delay to avoid 100% CPU on cRIO"
        # "UDP Broadcast loop"
        n200 = node-c288() -> (w313:T1)  [unwired: 4 in]
        n201 = String To IP(1:"239.1.4.6" ("name")) -> (0:w315:u32)
        n202 = call-poly <vilib>:"UDP Multicast Open.vi"("time-to-live (1)"=u16 5, "port"=u16 10001) -> ("error out"=w323:errorcluster, "connection ID"=w324:refnum<k16>)  [unwired: 8 in]
        n203 = timed-loop {
          tunnel: w324 -> [w344]
          tunnel: w323 -> [w343]
          tunnel: [w330] -> w319
          shift-right: [w333] -> _
          shift-left: FALSE -> [w336]
          tunnel: [w328] -> w317
          tunnel: w315 -> [w332]
          tunnel: u16 50001 ("port or service name") -> [w331]
          timing: w313 -> [_]
          timing-out: [_] -> w312
          tunnel: [w326] -> w311
          tunnel: w310 -> [w325]
          stop <- w327 stop-if-true
          n204 = node-c288() -> ()  [unwired: 1 in, 1 out]
          n205 = local read "Flight Number"() -> (w339:string)
          n206 = Select(t=FALSE, s=w336, f=TRUE) -> (s? t:f=w333:bool)
          "UDP packet \nstatus" <- w333
          n207 = feedback-in #2(w339) -> ()
          n208 = feedback #2() -> (w338:string)  [unwired: 1 in]
          n209 = Not Equal?(x=w339, y=w338) -> (x != y?=w337:bool)
          n210 = flat-sequence {
            tunnel: w332 -> [w352]
            tunnel: w343 -> [w353]
            tunnel: w344 -> [w354]
            tunnel: [w354] -> w342
            tunnel: [w353] -> w341
            tunnel: [w352] -> w340
            tunnel: w337 -> [w351]
            tunnel: w331 -> [w364]
            tunnel: w342 -> [w363]
            tunnel: w341 -> [w362]
            tunnel: w340 -> [w361]
            tunnel: [w360] -> w330
            tunnel: [w359] -> w328
            tunnel: w325 -> [w358]
            frame #0 {
              n211 = feedback #3(u32 0) -> (w348:u32)
              n212 = case shown="True" w351 {
                tunnel: w348 -> [w355 _]
                tunnel: [w355 u32 0] -> w347
                frame False {
                }
                frame True {
                }
              }
              "UDP_Pack_num" <- w347
              n213 = Increment(x=w347) -> (x+1=w349:u32)
              n214 = feedback-in #3(w349) -> ()
            }
            frame #1 {
              n215 = Dequeue Element(queue=w358) -> (element=w357:string)  [unwired: 2 in, 3 out]
              n216 = UDP Write(address=w361, port or service name=w364, connection ID=w363, data in=w357, 8:w362) -> (error out=w359:errorcluster, 3:w360:refnum<k16>)  [unwired: 1 in]
            }
          }
          n217 = local read "stop"() -> (w326:bool)
          n218 = Unbundle(w328) -> ("status"=w329:bool)  [unwired: 2 out]
          n219 = node-c288() -> ()  [unwired: 1 in, 1 out]
          n220 = Compound Arithmetic op=OR(w329, w326) -> (w327:bool)
        }
        n221 = Wait (ms)(milliseconds to wait=u32 1000) -> ()  [unwired: 1 out]
        n222 = node-c288(w312) -> ()  [unwired: 1 out]
        n223 = UDP Close(connection ID=w319, 8:w317) -> (error out=→"UDP_Out_Error":errorcluster)  [unwired: 1 out]
      }
      n224 = while {
        stop <- FALSE stop-if-true
        n225 = node-c288() -> (w254:T1)  [unwired: 4 in]
        n226 = Create Network Stream Reader Endpoint(7:10 ("reader buffer size"), 9:T4 {"Message"="", "Message Data"=variant} ("Message Cluster"), 11:"/command/reader/TEi43c" ("reader url")) -> (0:w260:errorcluster, 3:w261:refnum<k21>)  [unwired: 4 in]
        n227 = timed-loop "Host->Target Command Reader" {
          shift-right: [w271] -> w258
          shift-left: w260 -> [w274]
          shift-right: [w272] -> w257
          shift-left: w261 -> [w273]
          tunnel: [TRUE] -> _
          timing: w254 -> [_]
          timing-out: [_] -> w253
          stop <- w265 stop-if-true
          # "Receive Commands from Host VI"
          n228 = node-c288() -> ()  [unwired: 1 in, 1 out]
          n229 = shared-variable-read(w273, w274) -> (w272:refnum<k21>, w267:errorcluster, w269:bool, w270:T4)  [unwired: 1 in]
          n230 = Or(x=w269, y=w267) -> (x .or. y?=w268:bool)
          n231 = case shown="False" w268 {
            selector: w268 -> [_ w305]
            tunnel: w267 -> [w282 w306]
            tunnel: [w281 w306] -> w271
            tunnel: w270 -> [w279 _]
            tunnel: [w280 w305] -> w265
            frame False {
              n232 = Unbundle By Name(w279) -> ("Message"=w278:string, "Message Data"=w277:variant)
              n233 = case shown="\"V6\"" w278 {
                tunnel: w282 -> [w284 w288 w293 w299 w304]
                tunnel: [w284 w286 w292 w298 w303] -> w281
                tunnel: w277 -> [_ w289 w294 w297 w302]
                tunnel: [TRUE _ _ _ _] -> w280
                frame "Stop", Default {
                }
                frame "Stop File Write" {
                  n234 = Variant To Data(error in=w288, type=FALSE, Variant=w289) -> (data=→"Stop File Write":bool, error out=w286:errorcluster)
                }
                frame "UDP Time Offset" {
                  n235 = Variant To Data(error in=w293, type=0, Variant=w294) -> (data=→"UDP Time Stamp Offset":i32, error out=w292:errorcluster)
                }
                frame "V6" {
                  n236 = Variant To Data(error in=w299, type=FALSE, Variant=w297) -> (data=w295:bool, error out=w298:errorcluster)
                  "V6" <- w295
                  n237 = shared-variable "NI-cRIO9022-019C2C95\\Mod6\\DO4"(w295) -> ()  [unwired: 1 in, 1 out]
                }
                frame "Flight Number" {
                  n238 = Variant To Data(error in=w304, type="", Variant=w302) -> (data=→"Flight Number":string, error out=w303:errorcluster)
                }
              }
            }
            frame True {
            }
          }
          n239 = node-c288() -> ()  [unwired: 1 in, 1 out]
        }
        n240 = node-c288(w253) -> ()  [unwired: 1 out]
        n241 = Destroy Stream Endpoint(8:w258, 11:w257) -> (0:→"error out":errorcluster)
        n242 = Wait (ms)(milliseconds to wait=u32 1000) -> ()  [unwired: 1 out]
      }
      n243 = while {
        tunnel: w44 -> [w71]
        tunnel: w45 -> [w70]
        stop <- w74 stop-if-true
        # "Must delay to avoid 100% CPU on cRIO"
        # "TCP Loop writing to SEPTIC Tank"
        n244 = TCP Open Connection(address="192.168.101.108", remote port or service name=u16 3502) -> (connection ID=w77:refnum<k5>, error out=w72:errorcluster)  [unwired: 3 in]
        n245 = case shown="No Error" w72 {
          selector: w72 -> [w82 w109]
          tunnel: w77 -> [w87 w110]
          tunnel: [w86 w110] -> w76
          tunnel: [w85 w109] -> w75
          tunnel: [w84 w108] -> w74
          tunnel: w70 -> [w81 _]
          tunnel: w71 -> [w80 _]
          frame No Error {
            n246 = node-c288() -> (w89:T1)  [unwired: 4 in]
            n247 = timed-loop {
              tunnel: w87 -> [w103]
              tunnel: w82 -> [w102]
              tunnel: [w101] -> w86
              tunnel: [w100] -> w85
              tunnel: [w90] -> w84
              shift-right: [w94] -> _
              shift-left: FALSE -> [w97]
              timing: w89 -> [_]
              timing-out: [_] -> w88
              tunnel: w81 -> [w93]
              tunnel: w80 -> [w92]
              stop <- w98 stop-if-true
              n248 = node-c288() -> ()  [unwired: 1 in, 1 out]
              n249 = Dequeue Element(queue=w93, error in (no error)=w92) -> (element=w91:string)  [unwired: 1 in, 3 out]
              n250 = Select(t=FALSE, s=w97, f=TRUE) -> (s? t:f=w94:bool)
              "TCP packet\nSend to SEPTIC" <- w94
              n251 = TCP Write(connection ID=w103, data in=w91, error in (no error)=w102) -> (connection ID out=w101:refnum<k5>, error out=w100:errorcluster)  [unwired: 1 in, 1 out]
              n252 = local read "stop"() -> (w90:bool)
              n253 = Unbundle(w100) -> ("status"=w99:bool)  [unwired: 2 out]
              n254 = node-c288() -> ()  [unwired: 1 in, 1 out]
              n255 = Compound Arithmetic op=OR(w99, w90) -> (w98:bool)
            }
            n256 = node-c288(w88) -> ()  [unwired: 1 out]
          }
          frame Error {
            n257 = local read "stop"() -> (w108:bool)
          }
        }
        n258 = TCP Close Connection(connection ID=w76, error in (no error)=w75) -> (error out=→"SEPTIC TCP Error Out":errorcluster)  [unwired: 1 in, 1 out]
        n259 = Wait (ms)(milliseconds to wait=u32 1000) -> ()  [unwired: 1 out]
      }
      n260 = while {
        tunnel: w53 -> [w113]
        tunnel: w52 -> [w112]
        stop <- w116 stop-if-true
        # "Must delay to avoid 100% CPU on cRIO"
        # "TCP Loop writing to FISH Tank"
        n261 = TCP Open Connection(address="192.168.101.110", remote port or service name=u16 3502) -> (connection ID=w119:refnum<k5>, error out=w114:errorcluster)  [unwired: 3 in]
        n262 = case shown="No Error" w114 {
          selector: w114 -> [w124 w151]
          tunnel: w119 -> [w129 w152]
          tunnel: [w128 w152] -> w118
          tunnel: [w127 w151] -> w117
          tunnel: [w126 w150] -> w116
          tunnel: w113 -> [w123 _]
          tunnel: w112 -> [w122 _]
          frame No Error {
            n263 = node-c288() -> (w131:T1)  [unwired: 4 in]
            n264 = timed-loop {
              tunnel: w129 -> [w145]
              tunnel: w124 -> [w144]
              tunnel: [w143] -> w128
              tunnel: [w142] -> w127
              tunnel: [w139] -> w126
              shift-right: [w135] -> _
              shift-left: FALSE -> [w138]
              timing: w131 -> [_]
              timing-out: [_] -> w130
              tunnel: w123 -> [w134]
              tunnel: w122 -> [w133]
              stop <- w140 stop-if-true
              n265 = node-c288() -> ()  [unwired: 1 in, 1 out]
              n266 = Dequeue Element(queue=w134, error in (no error)=w133) -> (element=w132:string)  [unwired: 1 in, 3 out]
              n267 = Select(t=FALSE, s=w138, f=TRUE) -> (s? t:f=w135:bool)
              "TCP packet\nSend to FISH" <- w135
              n268 = TCP Write(connection ID=w145, data in=w132, error in (no error)=w144) -> (connection ID out=w143:refnum<k5>, error out=w142:errorcluster)  [unwired: 1 in, 1 out]
              n269 = local read "stop"() -> (w139:bool)
              n270 = Unbundle(w142) -> ("status"=w141:bool)  [unwired: 2 out]
              n271 = node-c288() -> ()  [unwired: 1 in, 1 out]
              n272 = Compound Arithmetic op=OR(w141, w139) -> (w140:bool)
            }
            n273 = node-c288(w130) -> ()  [unwired: 1 out]
          }
          frame Error {
            n274 = local read "stop"() -> (w150:bool)
          }
        }
        n275 = TCP Close Connection(connection ID=w118, error in (no error)=w117) -> (error out=→"FISH TCP Error Out":errorcluster)  [unwired: 1 in, 1 out]
        n276 = Wait (ms)(milliseconds to wait=u32 1000) -> ()  [unwired: 1 out]
      }
      n277 = node-c288(w39) -> ()  [unwired: 1 out]
    }
    frame Error {
    }
  }
  n278 = VISA Close(VISA resource name=w22, error in (no error)=w21) -> (error out=→"Serial Visa Error":errorcluster)
